vi "OSR_OSF.vi"(11 "BOOL":bool) -> (2 "OSF":bool, 3 "OSR":bool)   [LabVIEW 2018]
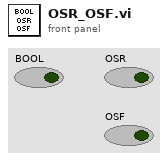
[diagram p1: front panel]
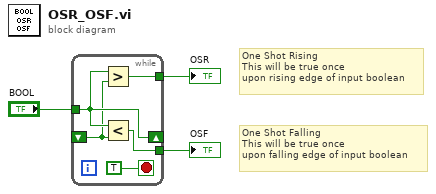
[diagram p0: block diagram]
diagram:
  # "One Shot Falling\nThis will be true once\nupon falling edge of input boolean"
  # "One Shot Rising\nThis will be true once\nupon rising edge of input boolean"
  n1 = while {
    shift-right: [w6] -> _
    shift-left: _ -> [w5]
    tunnel: "BOOL" -> [w6]
    tunnel: [w7] -> w2
    tunnel: [w4] -> w3
    stop <- TRUE stop-if-true
    n2 = Greater?(x=w6, y=w5) -> (0:w4:bool)
    n3 = Less?(x=w6, y=w5) -> (x < y?=w7:bool)
  }
  "OSR" <- w3
  "OSF" <- w2
